vi "WaitForConnectionProcess.vi"(0 "reference":refnum<class "VdTcpIP.lvclass">, 5 "error in (no error)":errorcluster) -> (14 "reference out":refnum<class "VdTcpIP.lvclass">, 19 "error out":errorcluster)   [LabVIEW 2020, in "VdTcpIP.lvclass"]
doc: "A backgroud process that handles incomming connections"
uses:
  VdTcpIP.lvclass
panel:
  # "VdTcpIp WaitForConnectionProccess"
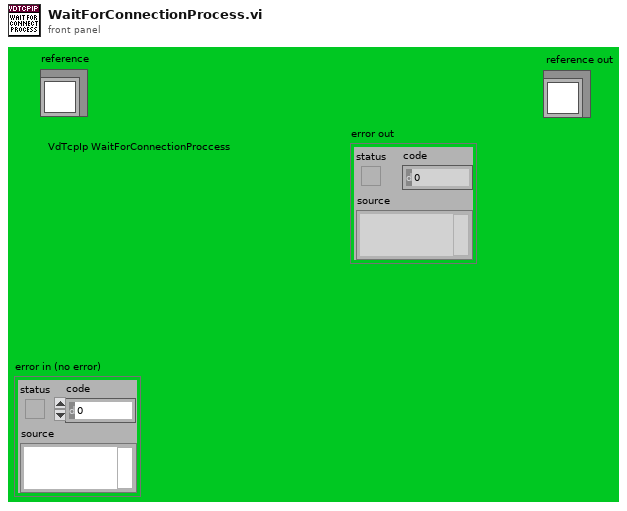
[diagram p1: front panel]
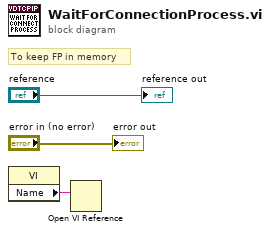
[diagram p0: block diagram]
diagram:
  # "To keep FP in memory"
  n1 = property class="VI"() -> ("Name"=w1:string)  [unwired: 2 in, 2 out]
  n2 = Open VI Reference(vi path=w1) -> ()  [unwired: 1 in, 6 out]
  "reference out" <- "reference"
  "error out" <- "error in (no error)"
